vi "K2400_V_lev.vi"(2 "error in":errorcluster, 3 "Voltage (V)":dbl format="%#_3g", 4 "address (24)":string) -> (0 "error out":errorcluster)   [LabVIEW 2021]
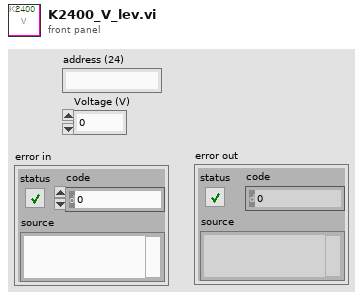
[diagram p1: front panel]
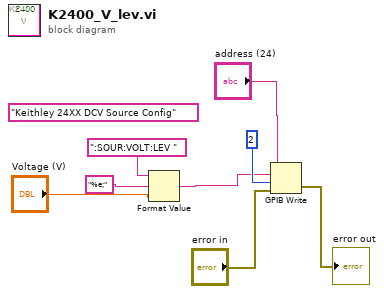
[diagram p0: block diagram]
diagram:
  (unwired) "Keithley 24XX DCV Source Config"
  n1 = Format Value(string ("")=":SOUR:VOLT:LEV ", format string="%e;", value (0)="Voltage (V)") -> (output string=w7:string)
  n2 = GPIB Write(0:"address (24)", 1:w7, 2:2, 3:"error in") -> (6:→"error out":errorcluster)  [unwired: 1 in, 1 out]
